vi "sendAddress.vi"(8 "error in (no error)":errorcluster, 10 "Address":i32, 11 "Mockbus in":refnum<class "Mockbus.lvclass">) -> (0 "error out":errorcluster, 3 "Mockbus out":refnum<class "Mockbus.lvclass">)   [LabVIEW 2015, in "RTMockbus.lvlib" / "Mockbus.lvclass"]
uses:
  Mockbus.lvclass
  Mockbus.lvclass/Mockbus.ctl
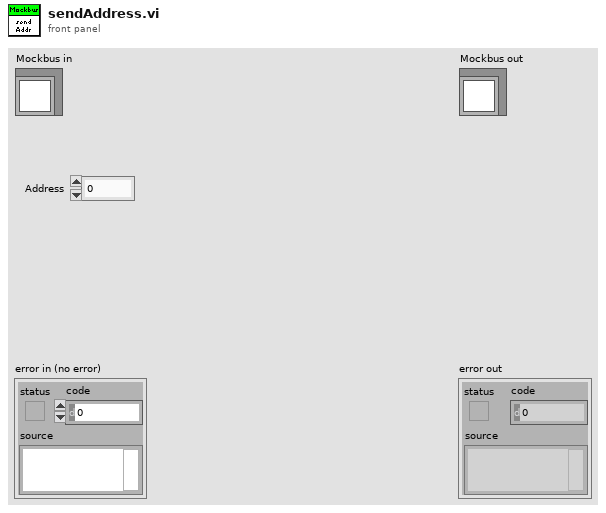
[diagram p1: front panel]
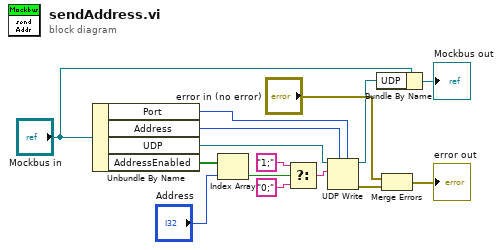
[diagram p0: block diagram]
diagram:
  n1 = Unbundle By Name("Mockbus in") -> ("Port"=w8:u16, "Address"=w9:u32, "UDP"=w10:refnum<k16>, "AddressEnabled"=w14:bool[])
  n2 = Index Array(array=w14, index="Address") -> (element=w13:bool)
  n3 = Select(t="1;", s=w13, f="0;") -> (s? t:f=w7:string)
  n4 = UDP Write(address=w9, port or service name=w8, connection ID=w10, data in=w7) -> (error out=w6:errorcluster, 3:w2:refnum<k16>)  [unwired: 2 in]
  n5 = Bundle By Name(cluster="Mockbus in", "UDP"=w2) -> (→"Mockbus out":refnum<class "Mockbus.lvclass">)
  n6 = Merge Errors("error in (no error)", w6) -> (→"error out":errorcluster)
